vi "Page_Source_Initialize.vi"(8 "error in (no error)":errorcluster, 9 "ctlReferences":T3, 11 "AB_RESTfulWebService in":refnum<class "AB_RESTfulWebService.lvclass">) -> (0 "error out":errorcluster, 1 "supportedFunctions":T1, 3 "AB_RESTfulWebService out":refnum<class "AB_RESTfulWebService.lvclass">)   [LabVIEW 2020, in "AB_RESTfulWebService.lvclass"]
uses:
  <vilib>/AppBuilder/AB_Classes/RESTful/AB_RESTfulWebService.lvclass
  <resource>/Framework/Providers/Builds/AppBuilder/AB_UI_Page_Source_Files_References.ctl
  <resource>/Framework/Providers/Builds/AppBuilder/AB_UI_Page_Source_Files_supportedFunctions.ctl
  <vilib>/AppBuilder/AB_Source_Inclusion.ctl
  <resource>/Framework/Providers/Common/provcom_StringGlobals.vi
  <vilib>/AppBuilder/AB_Classes/WebService/AB_WebService.lvclass
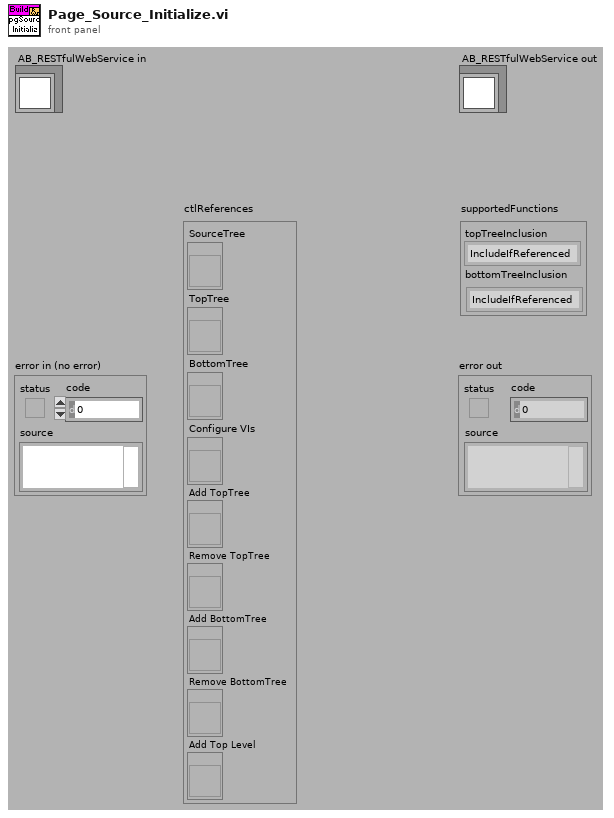
[diagram p1: front panel]
types:
  T1 = typedef "AB_UI_Page_Source_Files_supportedFunctions.ctl" = cluster{"topTreeInclusion":T2, "bottomTreeInclusion":T2}
  T2 = typedef "AB_Source_Inclusion.ctl" = enum16{"IncludeIfReferenced", "Include", "Exclude", "TopLevel"}
  T3 = typedef "AB_UI_Page_Source_Files_References.ctl" = cluster{"SourceTree":refnum<vi>, "TopTree":refnum<vi>, "BottomTree":refnum<vi>, "Configure VIs":refnum<vi>, "Add TopTree":refnum<vi>, "Remove TopTree":refnum<vi>, "Add BottomTree":refnum<vi>, "Remove BottomTree":refnum<vi>, "Add Top Level":refnum<vi>}
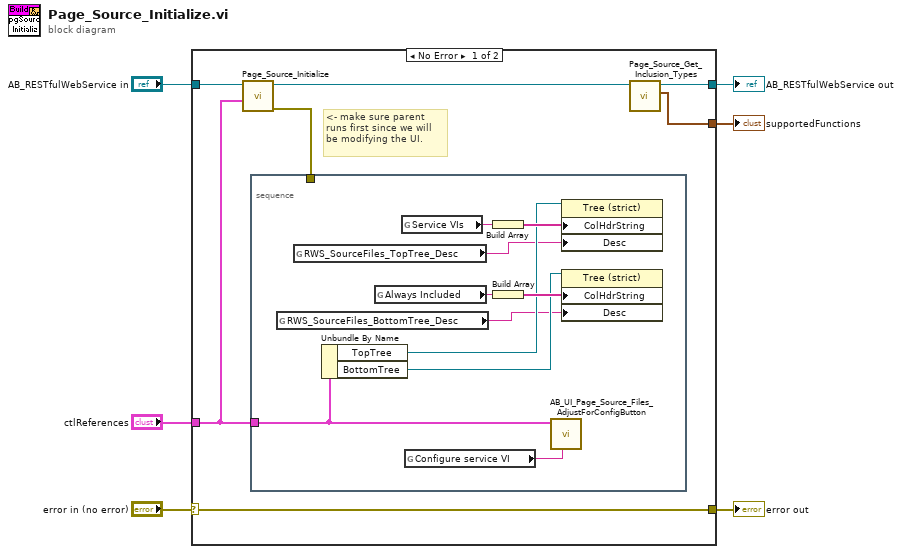
[diagram p0: block diagram]
diagram:
  n1 = case shown="No Error" "error in (no error)" {
    selector: "error in (no error)" -> [w13 w25]
    tunnel: [w13 w25] -> w2
    tunnel: "AB_RESTfulWebService in" -> [w10 w24]
    tunnel: "ctlReferences" -> [w8 _]
    tunnel: [w11 _] -> w4
    tunnel: [w12 w24] -> w5
    frame No Error {
      # "<- make sure parent runs first since we will be modifying the UI."
      n2 = call-parent "Page_Source_Initialize.vi"("ctlReferences"=w8, "AB_Build in"=w10) -> ("error out"=w7:errorcluster, "AB_Build out"=w9:refnum<class "AB_RESTfulWebService.lvclass">)  [unwired: 7 in, 1 out]
      n3 = stacked-sequence {
        tunnel: w8 -> [w14]
        tunnel: w7 -> [_]
        frame #0 {
          n4 = global read "provcom_StringGlobals.vi" "RWS_SourceFiles_BottomTree_Desc"() -> (w15:string)
          n5 = global read "provcom_StringGlobals.vi" "RWS_SourceFiles_TopTree_Desc"() -> (w16:string)
          n6 = Unbundle By Name(w14) -> ("TopTree"=w20:refnum<vi>, "BottomTree"=w19:refnum<vi>)
          n7 = global read "provcom_StringGlobals.vi" "Always Included"() -> (w23:string)
          n8 = global read "provcom_StringGlobals.vi" "Service VIs"() -> (w18:string)
          n9 = global read "provcom_StringGlobals.vi" "Configure service VI"() -> (w17:string)
          n10 = Build Array(w18) -> (w22:string[])
          n11 = Build Array(w23) -> (w21:string[])
          n12 = call <resource>:"AB_UI_Page_Source_Files_AdjustForConfigButton.vi"("config boolean string"=w17, "ctlReferences"=w14) -> ()  [unwired: 10 in]
          n13 = property class="Tree (strict)"(reference=w20, "ColHdrString"=w22, "Desc"=w16) -> ()  [unwired: 1 in, 2 out]
          n14 = property class="Tree (strict)"(reference=w19, "ColHdrString"=w21, "Desc"=w15) -> ()  [unwired: 1 in, 2 out]
        }
      }
      n15 = call-dynamic "Page_Source_Get_Inclusion_Types.vi"("AB_RESTfulWebService in"=w9) -> ("supportedFunctions"=w11:T1, "AB_RESTfulWebService out"=w12:refnum<class "AB_RESTfulWebService.lvclass">)  [unwired: 8 in, 1 out]
    }
    frame Error {
    }
  }
  "error out" <- w2
  "AB_RESTfulWebService out" <- w5
  "supportedFunctions" <- w4
